vi "Parent Check.vi"(8 "error in":errorcluster, 9 "Message Index":i32=-1, 10 "Parent Index":i32=-1, 11 "Message Data In":T1[](array[typedef])) -> (0 "error out":errorcluster, 2 "OK?":bool, 3 "Message Data Out":T1[](array[typedef]))   [LabVIEW 2020, in "SECS Communication.lvlib" / "SECS-II Class.lvclass"]
uses:
  SECS-II Class.lvclass
  Message Data.ctl
  Data Item Format.ctl
  Format Code.ctl
  SECS-II Class.lvclass/SECS-II Class.ctl
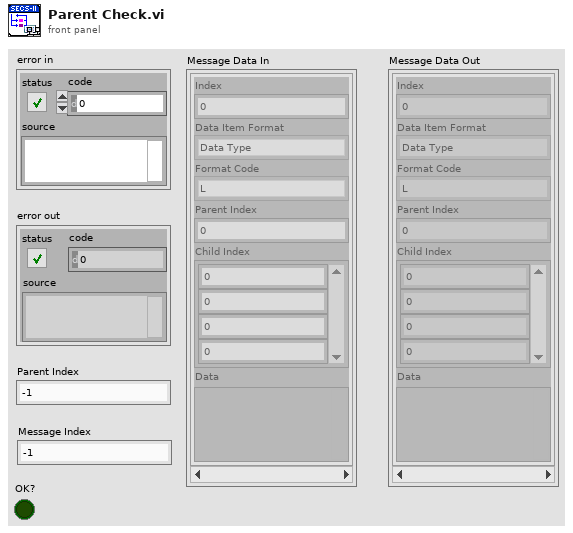
[diagram p1: front panel]
types:
  T1 = typedef "SECS Communication.lvlib/SECS-II Class.lvclass/Message Data.ctl" = cluster{"Index":i32, "Data Item Format":T2, "Format Code":T3, "Parent Index":i32, "Child Index":i32[], "Data":variant}
  T2 = typedef "SECS Communication.lvlib/SECS-II Class.lvclass/Data Item Format.ctl" = enum16{"Data Type", "Value"}
  T3 = typedef "SECS Communication.lvlib/SECS-II Class.lvclass/Format Code.ctl" = enum16{"L", "A", "B", "Boolean", "J", "I1", "I2", "I4", "I8", "U1", "U2", "U4", "U8", "F4", "F8", "Char"}
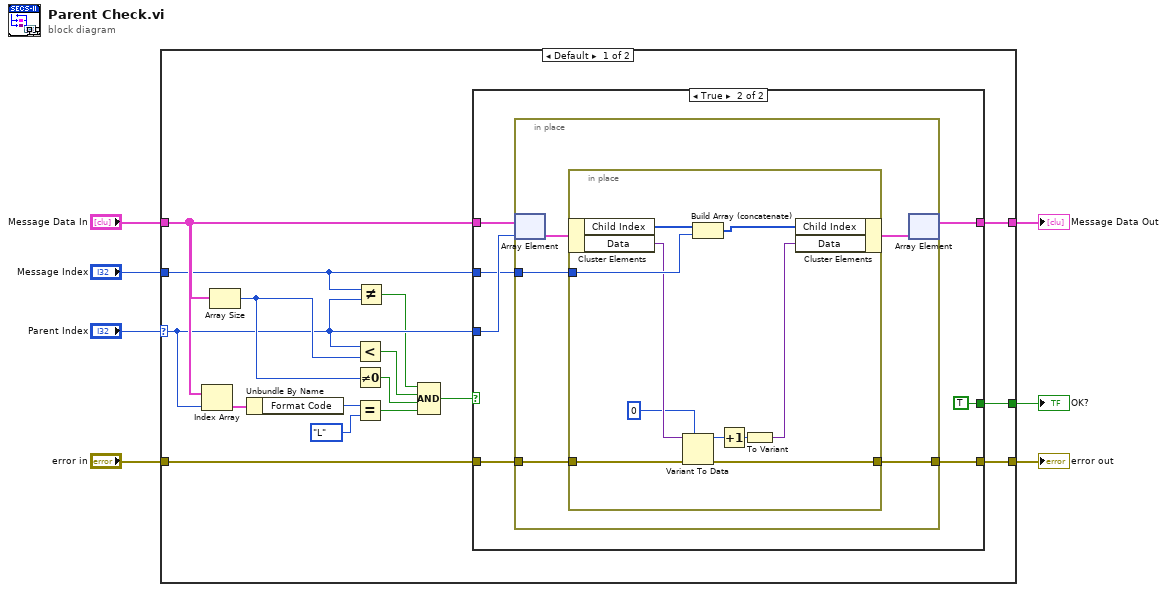
[diagram p0: block diagram]
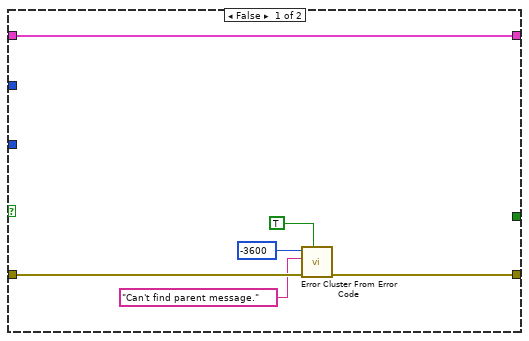
[diagram p2: hidden frame]
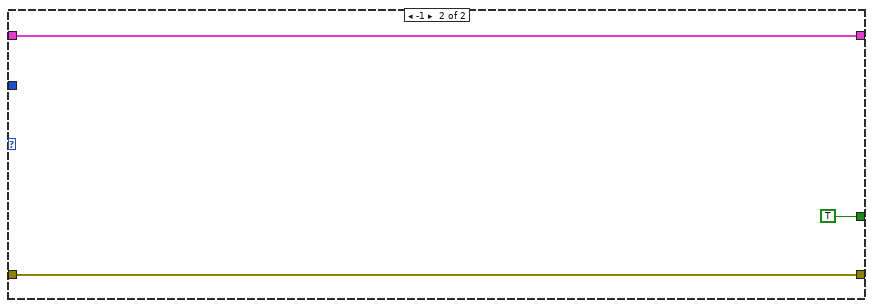
[diagram p3: hidden frame]
diagram:
  n1 = case shown="Default" "Parent Index" {
    selector: "Parent Index" -> [w11 _]
    tunnel: "Message Data In" -> [w21 w54]
    tunnel: "error in" -> [w22 w53]
    tunnel: [w18 w54] -> w5
    tunnel: [w17 w53] -> w4
    tunnel: [w8 TRUE] -> w3
    tunnel: "Message Index" -> [w9 _]
    frame Default {
      n2 = Index Array(array=w21, index=w11) -> (element=w23:T1)
      n3 = Array Size(array=w21) -> (size(s)=w13:i32)
      n4 = Unbundle By Name(w23) -> ("Format Code"=w20:T3)
      n5 = Less?(x=w11, y=w13) -> (x < y?=w12:bool)
      n6 = Not Equal To 0?(x=w13) -> (x != 0?=w15:bool)
      n7 = Equal?(x=w20, y=Format_Code."L") -> (x = y?=w16:bool)
      n8 = Not Equal?(x=w9, y=w11) -> (x != y?=w10:bool)
      n9 = Compound Arithmetic op=AND(w10, w12, w15, w16) -> (w14:bool)
      n10 = case shown="True" w14 {
        tunnel: w21 -> [w29 w36]
        tunnel: w22 -> [w28 w32]
        tunnel: w11 -> [_ w35]
        tunnel: [w29 w34] -> w18
        tunnel: [w27 w31] -> w17
        tunnel: w9 -> [_ w33]
        tunnel: [_ TRUE] -> w8
        frame False {
          n11 = call <vilib>:"Error Cluster From Error Code.vi"("show call chain? (False)"=TRUE, "error in (no error)"=w28, "error message (\"\")"="Can't find parent message." ("error message (\"\")"), "error code (0)"=-3600) -> ("error out"=w27:errorcluster)  [unwired: 5 in]
        }
        frame True {
          n12 = in-place {
            in-place-border: w33 -> [w39]
            in-place-border: w32 -> [w38]
            in-place-border: [w37] -> w31
            n13 = in-place-array #1(w36, w35) -> (w41:T1)
            n14 = in-place {
              in-place-border: w39 -> [w49]
              in-place-border: w38 -> [w48]
              in-place-border: [w42] -> w37
              n15 = in-place-cluster #2(w41) -> ("Child Index"=w51:i32[], "Data"=w47:variant)
              n16 = Variant To Data(error in=w48, type=0, Variant=w47) -> (data=w45:i32, error out=w42:errorcluster)
              n17 = Build Array (concatenate)(w51, w49) -> (w50:i32[])
              n18 = Increment(x=w45) -> (x+1=w44:i32)
              n19 = To Variant(anything=w44) -> (Variant=w43:variant)
              n20 = in-place-cluster #2("Child Index"=w50, "Data"=w43) -> (w40:T1)
            }
            n21 = in-place-array #1(w40) -> (w34:T1[])  [unwired: 1 out]
          }
        }
      }
    }
    frame -1 {
    }
  }
  "error out" <- w4
  "Message Data Out" <- w5
  "OK?" <- w3
